vi "unwrap data.vi"(10 "identifier":string, 11 "data to unwrap":string) -> (2 "unwrapped data":string, 3 "remaining string":string)   [LabVIEW 2025, in "CEF.lvlib" / "CEF_serializable configuration.lvclass"]
doc: "Parses a dataset of the following form:\n<identifier>data to wrap</identifier>Copyright 2017 National Instruments Corporation\n\nLicensed under the Apache License, Version 2.0 (the \"License\"); you may not use this file except in compliance with the License. You may obtain a copy of the License at http://www.apache.org/licenses/LICENSE-2.0\nUnless required by applicable law or agreed to in writing, software distributed under the License is distributed on an \"AS IS\" BASIS, WITHOUT WARRANTIES OR CONDITIONS OF ANY KIND, either express or implied. See the License for the specific language governing permissions and limitations under the License."
uses:
  CEF_serializable configuration.lvclass
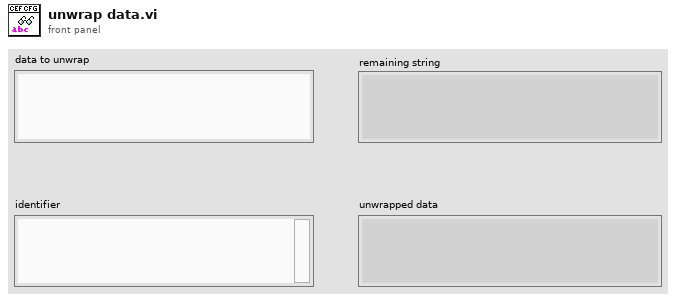
[diagram p1: front panel]
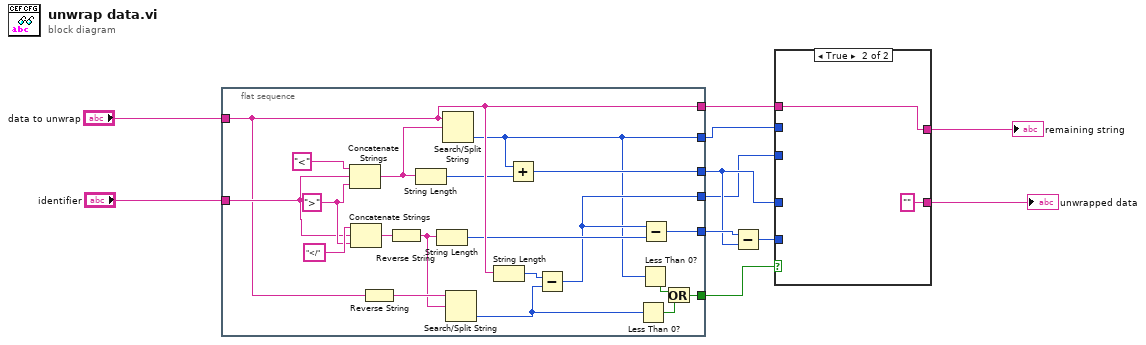
[diagram p0: block diagram]
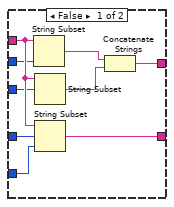
[diagram p2: hidden frame]
diagram:
  n1 = flat-sequence {
    tunnel: "identifier" -> [w28]
    tunnel: "data to unwrap" -> [w24]
    tunnel: [w15] -> w6
    tunnel: [w24] -> w7
    tunnel: [w21] -> w4
    tunnel: [w18] -> w5
    tunnel: [w17] -> w2
    tunnel: [w12] -> w1
    frame #0 {
      w29 = ">" ("string")
      n2 = Concatenate Strings("<" ("string"), w28, w29) -> (w23:string)
      n3 = Concatenate Strings("</" ("string"), w28, w29) -> (w27:string)
      n4 = Reverse String(1:w24) -> (0:w26:string)
      n5 = Reverse String(1:w27) -> (0:w20:string)
      n6 = String Length(string=w23) -> (length=w22:i32)
      n7 = String Length(string=w20) -> (length=w19:i32)
      n8 = Search/Split String(string=w24, search string/char (-)=w23) -> (offset of match=w15:i32)  [unwired: 1 in, 2 out]
      n9 = Search/Split String(string=w26, search string/char (-)=w20) -> (offset of match=w16:i32)  [unwired: 1 in, 2 out]
      n10 = String Length(string=w24) -> (length=w25:i32)
      n11 = Add(x=w15, y=w22) -> (x+y=w21:i32)
      n12 = Subtract(x=w25, y=w16) -> (x-y=w17:i32)
      n13 = Less Than 0?(x=w16) -> (x < 0?=w13:bool)
      n14 = Less Than 0?(x=w15) -> (x < 0?=w14:bool)
      n15 = Subtract(x=w17, y=w19) -> (x-y=w18:i32)
      n16 = Or(x=w14, y=w13) -> (x .or. y?=w12:bool)
    }
  }
  n17 = Subtract(x=w5, y=w4) -> (x-y=w3:i32)
  n18 = case shown="True" w1 {
    tunnel: [w40 w42] -> w9
    tunnel: [w39 "" ("data to unwrap")] -> w11
    tunnel: w7 -> [w36 w42]
    tunnel: w6 -> [w35 _]
    tunnel: w4 -> [w34 _]
    tunnel: w3 -> [w33 _]
    tunnel: w2 -> [w32 _]
    frame False {
      n19 = String Subset(string=w36, length (rest)=w35) -> (substring=w38:string)  [unwired: 1 in]
      n20 = String Subset(string=w36, offset (0)=w32) -> (substring=w37:string)  [unwired: 1 in]
      n21 = String Subset(string=w36, offset (0)=w34, length (rest)=w33) -> (substring=w39:string)
      n22 = Concatenate Strings(w38, w37) -> (w40:string)
    }
    frame True {
    }
  }
  "unwrapped data" <- w11
  "remaining string" <- w9
